vi "Cull and Group Peg.vi"(9 "Score Cutoff":dbl=3.0, 10 "Sorted Data":dbl[][](array[numeric])) -> (0 "Rect":T1, 1 "Line":T1, 2 "Score":dbl, 3 "Center":cluster{"X":dbl, "Y":dbl})   [LabVIEW 2016]
doc: "Examine the particle measurements to find the most likely pair that make up the target. This mostly compares the edges of the bounding boxes. It then returns information about the overall target, notably the rectangle sourrounding the particles, the vertical line that bisects the target, and the center of the top particle."
panel:
  out "Grouping Scores":T2(array[cluster])
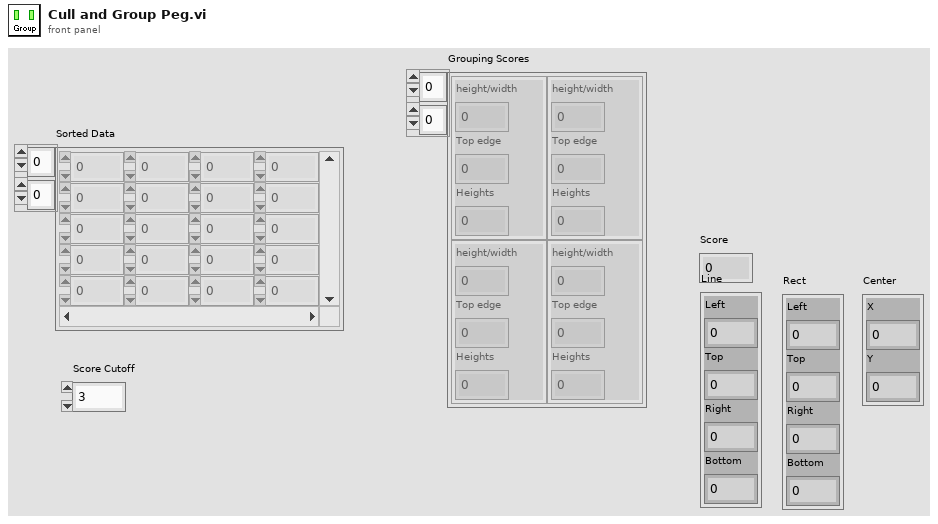
[diagram p1: front panel]
types:
  T1 = cluster{"Left":dbl, "Top":dbl, "Right":dbl, "Bottom":dbl}
  T2 = cluster{"height/width":dbl, "Top edge":dbl, "Heights":dbl}[][]
  T3 = cluster{"height/width":dbl, "Top edge":dbl, "Heights":dbl}
  T4 = cluster{"Left":dbl, "Numeric":dbl, "Right":dbl, "Numeric":dbl}
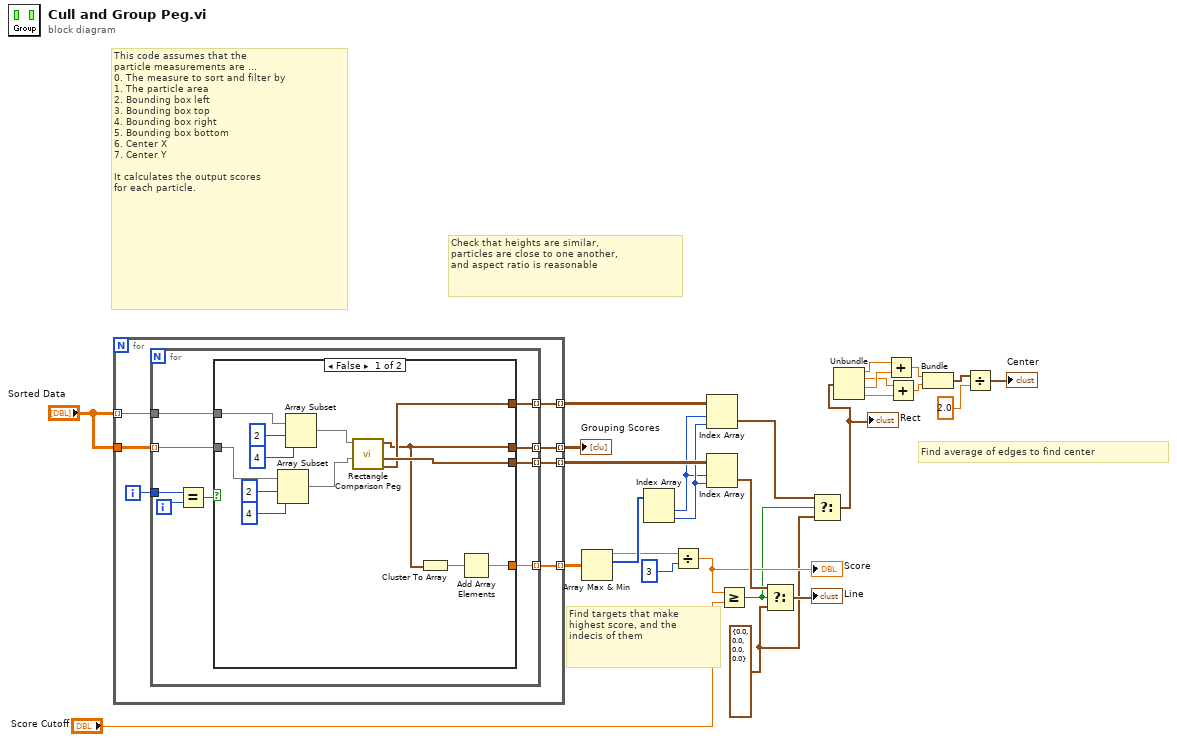
[diagram p0: block diagram]
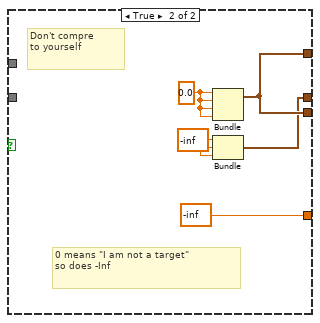
[diagram p2: hidden frame]
diagram:
  w4 = cluster{dbl, "Numeric":dbl, dbl, "Numeric":dbl} {0.0, "Numeric"=0.0, 0.0, "Numeric"=0.0} ("f")
  # "Find targets that make\nhighest score, and the\nindecis of them"
  # "Find average of edges to find center"
  # "Check that heights are similar,\nparticles are close to one another, \nand aspect ratio is reasonable"
  # "This code assumes that the\nparticle measurements are ...\n0. The measure to sort and filter by\n1. The particle area\n2. Bounding box left\n3. Bounding box top\n4. Bounding box right\n5. Bounding box bottom\n6. Center X\n7. Center Y\n\nIt calculates the output scores\nfor each particle."
  n1 = for {
    tunnel: "Sorted Data" -> [w34] mode=indexing
    tunnel: "Sorted Data" -> [w33]
    tunnel: [w31] -> w27 mode=indexing
    tunnel: [w30] -> w25 mode=indexing
    tunnel: [w29] -> w22 mode=indexing
    tunnel: [w28] -> w15 mode=indexing
    i -> [w32]
    n2 = for {
      tunnel: w34 -> [w43]
      tunnel: w33 -> [w41] mode=indexing
      tunnel: w32 -> [w40]
      tunnel: [w38] -> w31 mode=indexing
      tunnel: [w37] -> w30 mode=indexing
      tunnel: [w36] -> w29 mode=indexing
      tunnel: [w35] -> w28 mode=indexing
      i -> [w39]
      n3 = Equal?(x=w40, y=w39) -> (x = y?=w42:bool)
      n4 = case shown="False" w42 {
        tunnel: w43 -> [w54 _]
        tunnel: w41 -> [w51 _]
        tunnel: [w49 -inf] -> w38
        tunnel: [w46 w60] -> w37
        tunnel: [w45 w60] -> w36
        tunnel: [w44 w57] -> w35
        frame False {
          n5 = Array Subset(array=w51, index=2, length=4) -> (w48:dbl[])
          n6 = Array Subset(array=w54, index=2, length=4) -> (w47:dbl[])
          n7 = call "Rectangle Comparison Peg.vi"("Second"=w48, "First"=w47) -> ("Rect"=w45:T1, "Line"=w46:T1, "Scores"=w44:T3)  [unwired: 7 in]
          n8 = Cluster To Array(cluster=w44) -> (array=w50:dbl[])
          n9 = Add Array Elements(numeric array=w50) -> (sum=w49:dbl)
        }
        frame True {
          w58 = -inf
          w59 = 0.0
          # "0 means \"I am not a target\"\nso does -Inf"
          # "Don't compre\nto yourself"
          n10 = Bundle(w59, w59, w59, w59) -> (w60:cluster{dbl, dbl, dbl, dbl})  [unwired: 1 in]
          n11 = Bundle(w58, w58, w58) -> (w57:cluster{dbl, dbl, dbl})  [unwired: 1 in]
        }
      }
    }
  }
  "Grouping Scores" <- w15
  n12 = Array Max & Min(array=w27) -> (max value=w17:dbl, max index (indices)=w18:i32[])  [unwired: 2 out]
  n13 = Index Array(array=w18) -> (element #1=w19:i32, element #2=w21:i32)  [unwired: 2 in]
  n14 = Divide(x=w17, y=3 ("index")) -> (x/y=w16:dbl)
  "Score" <- w16
  n15 = Index Array(array=w22, index (row)=w19, index (col)=w21) -> (element=w2:T1)
  n16 = Index Array(array=w25, index (row)=w19, index (col)=w21) -> (element=w24:T1)
  n17 = Greater Or Equal?(x=w16, y="Score Cutoff") -> (x >= y?=w3:bool)
  n18 = Select(t=w24, s=w3, f=w4) -> (s? t:f=→"Line":T4)
  n19 = Select(t=w2, s=w3, f=w4) -> (s? t:f=w1:T4)
  "Rect" <- w1
  n20 = Unbundle(w1) -> ("Left"=w14:dbl, "Numeric"=w6:dbl, "Right"=w13:dbl, "Numeric"=w11:dbl)
  n21 = Add(x=w14, y=w13) -> (x+y=w12:dbl)
  n22 = Add(x=w6, y=w11) -> (x+y=w10:dbl)
  n23 = Bundle(w12, w10) -> (w9:cluster{dbl, dbl})  [unwired: 1 in]
  n24 = Divide(x=w9, y=2.0) -> (x/y=→"Center":cluster{dbl, dbl})
